vi "SDL Renderer Present.vi"(8 "error in (no error)":errorcluster) -> (0 "error out":errorcluster)   [LabVIEW 2021, in "Main Controller Actor.lvclass"]
uses:
  Main Controller Actor.lvclass
  LabSDL2/Source/Libraries/LibSDL2 Wrapper/LibSDL2.lvlib
  Globals.vi
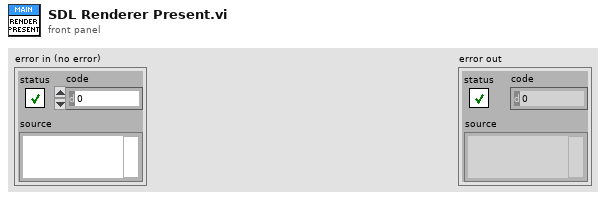
[diagram p1: front panel]
types:
  T1 = cluster{"Renderer":u32, "Font":u32, "Window":u32, "Joystick":u32}
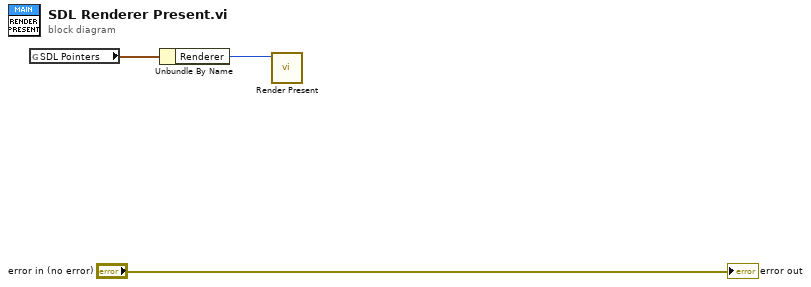
[diagram p0: block diagram]
diagram:
  n1 = global read "Globals.vi" "SDL Pointers"() -> (w1:T1)
  n2 = Unbundle By Name(w1) -> ("Renderer"=w2:u32)
  n3 = call "Render Present.vi"("Renderer Pointer"=w2) -> ()  [unwired: 10 in, 1 out]
  "error out" <- "error in (no error)"
